vi "FPGAtester2.vi"() -> ()   [LabVIEW 2013]
uses:
  <vilib>/DAQmx/read.llb/DAQmx Read (Counter DBL 1Chan 1Samp).vi
  <vilib>/DAQmx/write.llb/DAQmx Write (Digital Bool 1Line 1Point).vi
  <vilib>/DAQmx/read.llb/DAQmx Read (Digital Bool 1Line 1Point).vi
  <vilib>/Utility/file.llb/Read From Spreadsheet File (I64).vi
  <vilib>/DAQmx/create/channels.llb/DAQmx Create Channel (CI-Pulse Width).vi
  <vilib>/DAQmx/miscellaneous.llb/DAQmx Fill In Error Info.vi
  <vilib>/Utility/file.llb/Write To Spreadsheet File (DBL).vi
panel:
  out "Error out":errorcluster[][](array[cluster])
  in  "Delay":u32
  in  "error in":errorcluster
  in  "GPIB address":string="15"
  in  "Write to file?":bool
  out "Trial time vs. photons counted":cluster{"Y":dbl[], "Y":dbl[]}[](graph)
  out "Results":dbl[][](array[numeric])
  out "all rows":i64[][](array[numeric])
  in  "Read Excel file?":bool
  out "Current level":u16
  in  "Repetitions":dbl=1.0
  in  "Levels":i16[](array[numeric])
  out "Set 1":bool[](array[boolean])
  out "Set 2":bool[](array[boolean])
  out "Set 3":bool[](array[boolean])
  out "Set 4":bool[](array[boolean])
  out "16-bit number":bool[](array[boolean])
  # "Or specify levels below:"
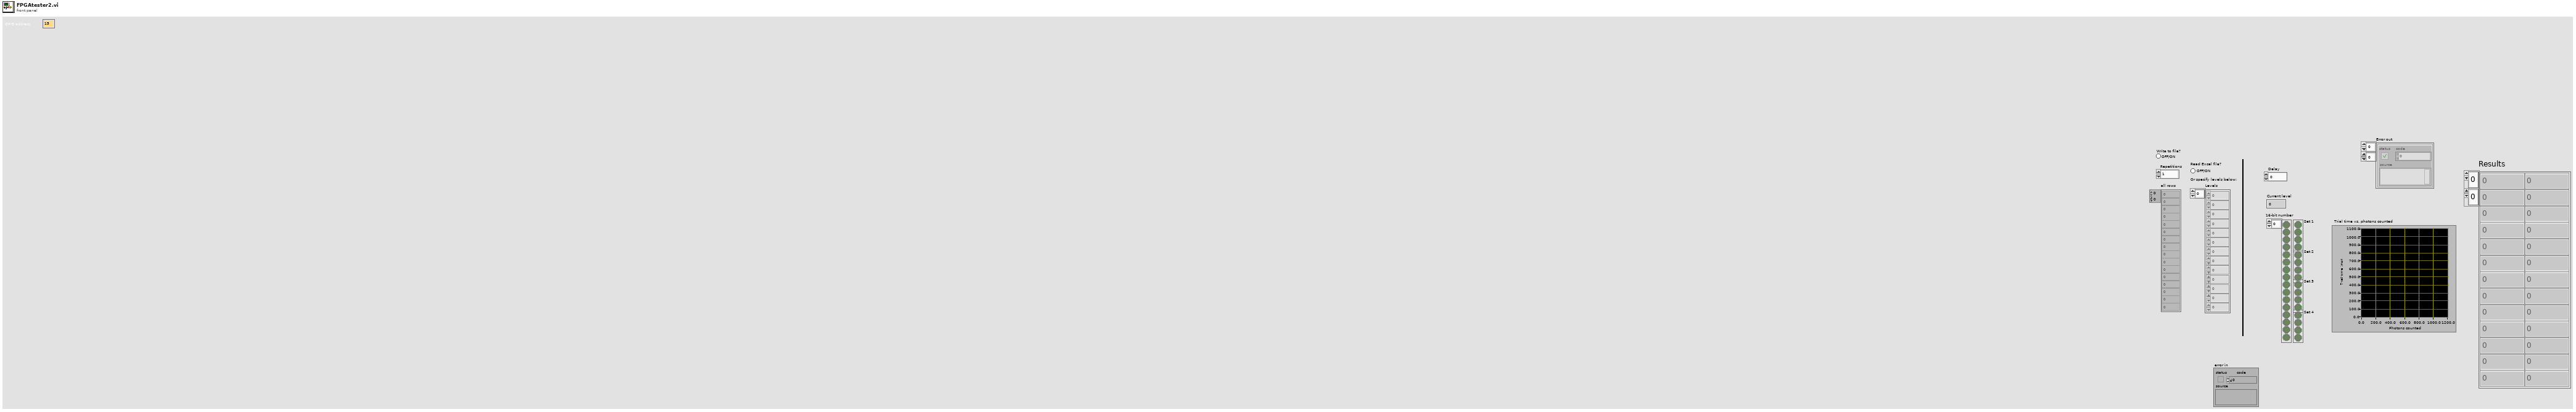
[diagram p1: front panel]
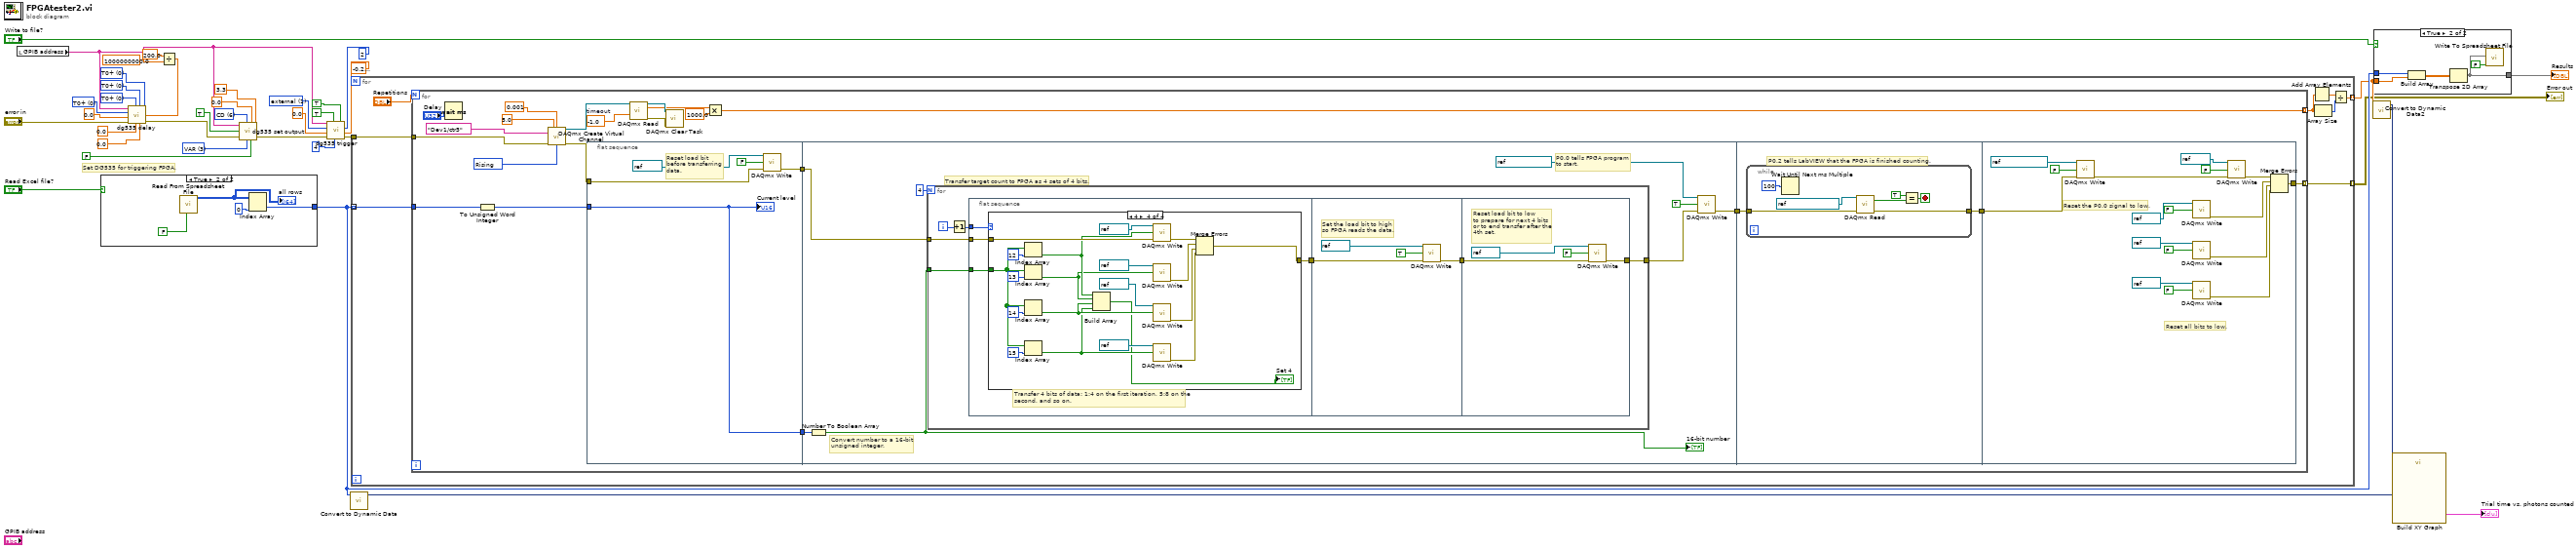
[diagram p0: block diagram]
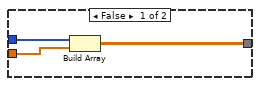
[diagram p2: hidden frame]
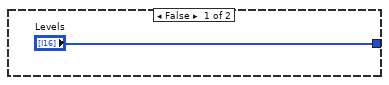
[diagram p3: hidden frame]
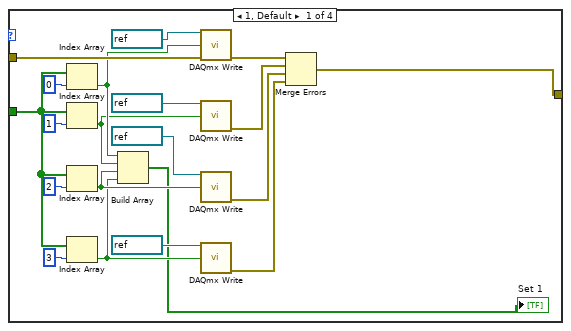
[diagram p4: hidden frame]
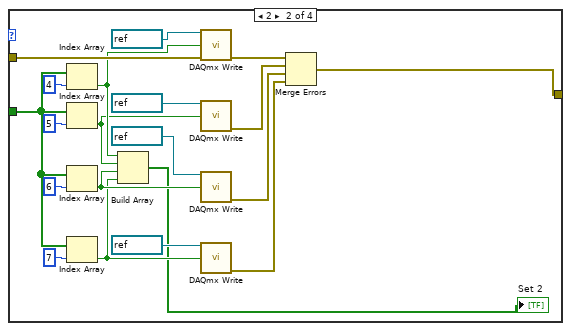
[diagram p5: hidden frame]
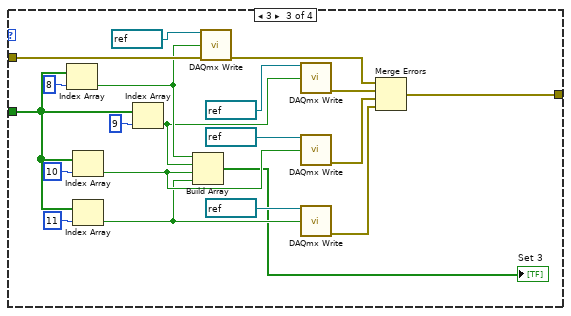
[diagram p6: hidden frame]
diagram:
  w18 = u32 1 items=["internal", "external", "single shot", "burst", "line"] ("trigger")
  w20 = 3 items=["TTL", "NIM", "ECL", "VAR"] ("mode")
  w22 = u16 6 items=["T0", "A", "B", "AB", "C", "D", "CD"] ("output")
  w25 = u32 0 items=["T0+", "A+", "B+", "C+"] ("D=")
  w26 = u32 0 items=["T0+", "A+", "B+", "D+"] ("C=")
  w27 = u32 0 items=["T0+", "A+", "C+", "D+"] ("B=")
  w28 = u32 0 items=["T0+", "B+", "C+", "D+"] ("A=")
  # "Set DG535 for triggering FPGA."
  n1 = local read "GPIB address"() -> (w10:string)
  n2 = case shown="True" "Read Excel file?" {
    tunnel: ["Levels" w41] -> w35
    frame False {
    }
    frame True {
      n3 = call-poly <vilib>:"Read From Spreadsheet File.vi"("transpose (no:F)"=FALSE) -> ("all rows"=w42:i64[][])  [unwired: 6 in, 4 out]
      "all rows" <- w42
      n4 = Index Array(array=w42, index (col)=0 ("disabled index (col)")) -> (element=w41:i64[])  [unwired: 1 in]
    }
  }
  n5 = Divide(x=200.0 ("D"), y=1000000000.0) -> (x/y=w4:dbl)
  n6 = call "dg535 delay.vi"("C"=0.0, "D"=w4, "D="=w25, "C="=w26, "B"=0.0 ("C"), "error in"="error in", "A"=0.0 ("D"), "B="=w27, "A="=w28, "GPIB address"=w10) -> ("error out"=w24:errorcluster)
  n7 = call "dg535 set output.vi"("GPIB address"=w10, "output"=w22, "set"=TRUE, "error in"=w24, "mode"=w20, "offset"=0.0, "amplitude"=3.3, "load"=FALSE) -> ("error out"=w11:errorcluster)  [unwired: 1 in]
  n8 = call "dg535 trigger.vi"("external trigger level"=sgl -0.2, "burst count"=2, "trigger slope"=TRUE, "burst period"=4, "input impedance"=TRUE, "error in"=w11, "internal/burst trigger rate"=0.0, "trigger"=w18, "GPIB address"=w10) -> ("error out"=w3:errorcluster)
  n9 = call "Convert to Dynamic Data"("Array"=w35) -> ("Dynamic Data Type"=w34:dynamicdata)  [unwired: 3 in]
  n10 = for {
    tunnel: w35 -> [w49] mode=indexing
    tunnel: [w45] -> w33 mode=indexing
    tunnel: w3 -> [w44]
    tunnel: [w43] -> w1 mode=indexing
    n11 = for {
      N: "Repetitions" -> [_]
      tunnel: w49 -> [w56]
      tunnel: [w55] -> w46 mode=indexing
      tunnel: w44 -> [w53]
      tunnel: [w51] -> w43 mode=indexing
      w60 = -1.0  # timeout
      w63 = 10280 items=["Rising"=10280, "Falling"=10171] ("Starting Edge")
      n12 = Wait (ms)(milliseconds to wait="Delay") -> ()  [unwired: 1 out]
      n13 = To Unsigned Word Integer(number=w56) -> (unsigned 16bit integer=w67:u16)
      n14 = call-poly <vilib>:"DAQmx Create Virtual Channel.vi"("maximum value"=5.0 ("Maximum Value (sec)"), "minimum value"=0.001 ("Minimum Value (sec)"), "counter"=tag "Dev1/ctr3" ("Physical Channel"), "error in"=w53, "starting edge"=w63) -> ("task out"=w54:refnum<k21>, "error out"=w57:errorcluster)  [unwired: 9 in]
      n15 = flat-sequence {
        tunnel: w57 -> [w73]
        tunnel: w67 -> [w76]
        tunnel: [w76] -> w71
        tunnel: [w72] -> w70
        tunnel: [w77] -> w69
        tunnel: w71 -> [w84]
        tunnel: w70 -> [w81]
        tunnel: w69 -> [w185]
        tunnel: [w184] -> w68
        tunnel: [w193] -> w51
        tunnel: w68 -> [w199]
        frame #0 {
          # "Reset load bit\nbefore transferring\ndata."
          n16 = call-poly <vilib>:"DAQmx Write.vi"("task/channels in"=refnum<k21> "BIT5", "data"=FALSE, "error in"=w73) -> ("error out"=w72:errorcluster)  [unwired: 10 in, 2 out]
          "Current level" <- w76
        }
        frame #1 {
          # "P0.0 tells FPGA program \nto start."
          # "Convert number to a 16-bit\nunsigned integer."
          # "Transfer target count to FPGA as 4 sets of 4 bits."
          n17 = Number To Boolean Array(number=w84) -> (Boolean array=w82:bool[])
          "16-bit number" <- w82
          n18 = for {
            N: 4 -> [_]
            tunnel: w82 -> [w88]
            tunnel: w81 -> [w90]
            tunnel: [w85] -> w78
            i -> [w91]
            n19 = Increment(x=w91) -> (x+1=w89:i32)
            n20 = flat-sequence {
              tunnel: w90 -> [w95]
              tunnel: w89 -> [w94]
              tunnel: w88 -> [w93]
              tunnel: [w92] -> w87
              tunnel: w87 -> [w177]
              tunnel: [w176] -> w86
              tunnel: w86 -> [w181]
              tunnel: [w180] -> w85
              frame #0 {
                # "Transfer 4 bits of data: 1:4 on the first iteration, 5:8 on the\nsecond, and so on."
                n21 = case shown="4" w94 {
                  tunnel: w93 -> [w103 w123 w143 w163]
                  tunnel: w95 -> [w102 w122 w142 w162]
                  tunnel: [w101 w121 w141 w161] -> w92
                  frame 1, Default {
                    n22 = Index Array(array=w103, index=0) -> (element=w100:bool)
                    n23 = Index Array(array=w103, index=1) -> (element=w99:bool)
                    n24 = Index Array(array=w103, index=2) -> (element=w98:bool)
                    n25 = Index Array(array=w103, index=3) -> (element=w97:bool)
                    n26 = Build Array(w100, w99, w98, w97) -> (→"Set 1":bool[])
                    n27 = call-poly <vilib>:"DAQmx Write.vi"("task/channels in"=refnum<k21> "BIT1", "data"=w100, "error in"=w102) -> ("error out"=w111:errorcluster)  [unwired: 10 in, 2 out]
                    n28 = call-poly <vilib>:"DAQmx Write.vi"("task/channels in"=refnum<k21> "BIT2", "data"=w99) -> ("error out"=w110:errorcluster)  [unwired: 11 in, 2 out]
                    n29 = call-poly <vilib>:"DAQmx Write.vi"("task/channels in"=refnum<k21> "BIT3", "data"=w98) -> ("error out"=w109:errorcluster)  [unwired: 11 in, 2 out]
                    n30 = call-poly <vilib>:"DAQmx Write.vi"("task/channels in"=refnum<k21> "BIT4", "data"=w97) -> ("error out"=w108:errorcluster)  [unwired: 11 in, 2 out]
                    n31 = Merge Errors(w111, w110, w109, w108) -> (w101:errorcluster)
                  }
                  frame 2 {
                    n32 = Index Array(array=w123, index=4) -> (element=w120:bool)
                    n33 = Index Array(array=w123, index=5) -> (element=w119:bool)
                    n34 = Index Array(array=w123, index=6) -> (element=w118:bool)
                    n35 = Index Array(array=w123, index=7) -> (element=w117:bool)
                    n36 = Build Array(w120, w119, w118, w117) -> (→"Set 2":bool[])
                    n37 = call-poly <vilib>:"DAQmx Write.vi"("task/channels in"=refnum<k21> "BIT1", "data"=w120, "error in"=w122) -> ("error out"=w131:errorcluster)  [unwired: 10 in, 2 out]
                    n38 = call-poly <vilib>:"DAQmx Write.vi"("task/channels in"=refnum<k21> "BIT2", "data"=w119) -> ("error out"=w130:errorcluster)  [unwired: 11 in, 2 out]
                    n39 = call-poly <vilib>:"DAQmx Write.vi"("task/channels in"=refnum<k21> "BIT3", "data"=w118) -> ("error out"=w129:errorcluster)  [unwired: 11 in, 2 out]
                    n40 = call-poly <vilib>:"DAQmx Write.vi"("task/channels in"=refnum<k21> "BIT4", "data"=w117) -> ("error out"=w128:errorcluster)  [unwired: 11 in, 2 out]
                    n41 = Merge Errors(w131, w130, w129, w128) -> (w121:errorcluster)
                  }
                  frame 3 {
                    n42 = Index Array(array=w143, index=8) -> (element=w140:bool)
                    n43 = Index Array(array=w143, index=10) -> (element=w138:bool)
                    n44 = Index Array(array=w143, index=11) -> (element=w137:bool)
                    n45 = Index Array(array=w143, index=9) -> (element=w139:bool)
                    n46 = Build Array(w140, w139, w138, w137) -> (→"Set 3":bool[])
                    n47 = call-poly <vilib>:"DAQmx Write.vi"("task/channels in"=refnum<k21> "BIT1", "data"=w140, "error in"=w142) -> ("error out"=w151:errorcluster)  [unwired: 10 in, 2 out]
                    n48 = call-poly <vilib>:"DAQmx Write.vi"("task/channels in"=refnum<k21> "BIT2", "data"=w139) -> ("error out"=w150:errorcluster)  [unwired: 11 in, 2 out]
                    n49 = call-poly <vilib>:"DAQmx Write.vi"("task/channels in"=refnum<k21> "BIT3", "data"=w138) -> ("error out"=w149:errorcluster)  [unwired: 11 in, 2 out]
                    n50 = call-poly <vilib>:"DAQmx Write.vi"("task/channels in"=refnum<k21> "BIT4", "data"=w137) -> ("error out"=w148:errorcluster)  [unwired: 11 in, 2 out]
                    n51 = Merge Errors(w151, w150, w149, w148) -> (w141:errorcluster)
                  }
                  frame 4 {
                    n52 = Index Array(array=w163, index=12) -> (element=w160:bool)
                    n53 = Index Array(array=w163, index=13) -> (element=w159:bool)
                    n54 = Index Array(array=w163, index=14) -> (element=w158:bool)
                    n55 = Index Array(array=w163, index=15) -> (element=w157:bool)
                    n56 = Build Array(w160, w159, w158, w157) -> (→"Set 4":bool[])
                    n57 = call-poly <vilib>:"DAQmx Write.vi"("task/channels in"=refnum<k21> "BIT1", "data"=w160, "error in"=w162) -> ("error out"=w171:errorcluster)  [unwired: 10 in, 2 out]
                    n58 = call-poly <vilib>:"DAQmx Write.vi"("task/channels in"=refnum<k21> "BIT2", "data"=w159) -> ("error out"=w170:errorcluster)  [unwired: 11 in, 2 out]
                    n59 = call-poly <vilib>:"DAQmx Write.vi"("task/channels in"=refnum<k21> "BIT3", "data"=w158) -> ("error out"=w169:errorcluster)  [unwired: 11 in, 2 out]
                    n60 = call-poly <vilib>:"DAQmx Write.vi"("task/channels in"=refnum<k21> "BIT4", "data"=w157) -> ("error out"=w168:errorcluster)  [unwired: 11 in, 2 out]
                    n61 = Merge Errors(w171, w170, w169, w168) -> (w161:errorcluster)
                  }
                }
              }
              frame #1 {
                # "Set the load bit to high\nso FPGA reads the data."
                n62 = call-poly <vilib>:"DAQmx Write.vi"("task/channels in"=refnum<k21> "BIT5", "data"=TRUE, "error in"=w177) -> ("error out"=w176:errorcluster)  [unwired: 10 in, 2 out]
              }
              frame #2 {
                # "Reset load bit to low\nto prepare for next 4 bits\nor to end transfer after the\n4th set."
                n63 = call-poly <vilib>:"DAQmx Write.vi"("task/channels in"=refnum<k21> "BIT5", "data"=FALSE, "error in"=w181) -> ("error out"=w180:errorcluster)  [unwired: 10 in, 2 out]
              }
            }
          }
          n64 = call-poly <vilib>:"DAQmx Write.vi"("task/channels in"=refnum<k21> "LaserChannel", "data"=TRUE, "error in"=w78) -> ("error out"=w77:errorcluster)  [unwired: 10 in, 2 out]
        }
        frame #2 {
          # "P0.2 tells LabVIEW that the FPGA is finished counting."
          n65 = while {
            tunnel: w185 -> [w191]
            tunnel: [w190] -> w184
            stop <- w187 stop-if-true
            n66 = Wait Until Next ms Multiple(millisecond multiple=u32 100) -> ()  [unwired: 1 out]
            n67 = call-poly <vilib>:"DAQmx Read.vi"("task/channels in"=refnum<k21> "P02countSignal", "error in"=w191) -> ("data"=w188:bool, "error out"=w190:errorcluster)  [unwired: 11 in, 1 out]
            n68 = Equal?(x=TRUE, y=w188) -> (x = y?=w187:bool)
          }
        }
        frame #3 {
          # "Reset all bits to low."
          # "Reset the P0.0 signal to low."
          n69 = call-poly <vilib>:"DAQmx Write.vi"("task/channels in"=refnum<k21> "LaserChannel", "data"=FALSE, "error in"=w199) -> ("error out"=w198:errorcluster)  [unwired: 10 in, 2 out]
          n70 = call-poly <vilib>:"DAQmx Write.vi"("task/channels in"=refnum<k21> "BIT2", "data"=FALSE) -> ("error out"=w206:errorcluster)  [unwired: 11 in, 2 out]
          n71 = call-poly <vilib>:"DAQmx Write.vi"("task/channels in"=refnum<k21> "BIT3", "data"=FALSE) -> ("error out"=w205:errorcluster)  [unwired: 11 in, 2 out]
          n72 = call-poly <vilib>:"DAQmx Write.vi"("task/channels in"=refnum<k21> "BIT4", "data"=FALSE) -> ("error out"=w204:errorcluster)  [unwired: 11 in, 2 out]
          n73 = call-poly <vilib>:"DAQmx Write.vi"("task/channels in"=refnum<k21> "BIT1", "data"=FALSE, "error in"=w198) -> ("error out"=w207:errorcluster)  [unwired: 10 in, 2 out]
          n74 = Merge Errors(w207, w206, w205, w204) -> (w193:errorcluster)
        }
      }
      n75 = call-poly <vilib>:"DAQmx Read.vi"("task/channels in"=w54, "timeout"=w60) -> ("task out"=w62:refnum<k21>, "data"=w58:dbl, "error out"=w61:errorcluster)  [unwired: 11 in]
      n76 = call <vilib>:"DAQmx Clear Task.vi"("task in"=w62, "error in"=w61) -> ()  [unwired: 13 in, 1 out]
      n77 = Multiply(x=w58, y=1000.0) -> (x*y=w55:dbl)
    }
    n78 = Add Array Elements(numeric array=w46) -> (sum=w48:dbl)
    n79 = Array Size(array=w46) -> (size(s)=w47:i32)
    n80 = Divide(x=w48, y=w47) -> (x/y=w45:dbl)
  }
  "Error out" <- w1
  n81 = call "Convert to Dynamic Data2"("Array"=w33) -> ("Dynamic Data Type"=w32:dynamicdata)  [unwired: 3 in]
  n82 = case shown="True" "Write to file?" {
    tunnel: w33 -> [w211 w217]
    tunnel: w35 -> [w212 w216]
    tunnel: [w210 w213] -> w30
    frame False {
      n83 = Build Array(w212, w211) -> (w210:dbl[][])
    }
    frame True {
      n84 = Build Array(w216, w217) -> (w214:dbl[][])
      n85 = Transpose 2D Array(2D array=w214) -> (transposed array=w213:dbl[][])
      n86 = call-poly <vilib>:"Write To Spreadsheet File.vi"("append to file? (new file:F)"=FALSE, "2D data"=w213) -> ()  [unwired: 6 in, 1 out]
    }
  }
  "Results" <- w30
  n87 = call "Build XY Graph"("Y Input"=w32, "X Input"=w34) -> ("XY Graph"=→"Trial time vs. photons counted":cluster{"Y":dbl[], "Y":dbl[]}[])  [unwired: 3 in, 6 out]
